vi "Split UDP Data Array.vi"(0 "Array in":string[][](array[string])) -> (1 "Column 1":string[](array[string]), 2 "Column 2":string[](array[string]), 3 "Column 3":string[](array[string]), 4 "Column 4":string[](array[string]))   [LabVIEW 2017]
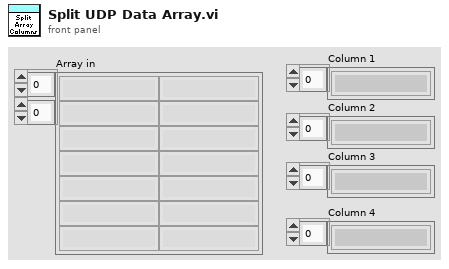
[diagram p1: front panel]
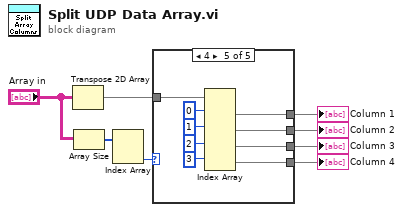
[diagram p0: block diagram]
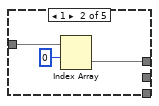
[diagram p3: hidden frame]
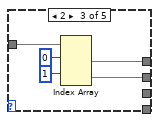
[diagram p4: hidden frame]
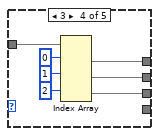
[diagram p5: hidden frame]
diagram:
  n1 = Transpose 2D Array(2D array="Array in") -> (transposed array=w8:string[][])
  n2 = Array Size(array="Array in") -> (size(s)=w6:i32[])
  n3 = Index Array(array=w6) -> (element #2=w5:i32)  [unwired: 2 in, 1 out]
  n4 = case shown="4" w5 {
    tunnel: w8 -> [_ w11 w16 w23 w32]
    tunnel: [_ _ _ _ w27] -> w1
    tunnel: [_ _ _ w17 w26] -> w2
    tunnel: [_ _ w12 w18 w25] -> w3
    tunnel: [_ w9 w13 w19 w24] -> w4
    frame Default {
    }
    frame 1 {
      n5 = Index Array(array=w11, index (row)=0) -> (element=w9:string[])  [unwired: 1 in]
    }
    frame 2 {
      n6 = Index Array(array=w16, index (row) #1=0 ("index (row)"), index (row) #2=1 ("index (row)")) -> (element #1=w13:string[], element #2=w12:string[])  [unwired: 2 in]
    }
    frame 3 {
      n7 = Index Array(array=w23, index (row) #1=0 ("index (row)"), index (row) #2=1 ("index (row)"), index (row) #3=2 ("index (row)")) -> (element #1=w19:string[], element #2=w18:string[], element #3=w17:string[])  [unwired: 3 in]
    }
    frame 4 {
      n8 = Index Array(array=w32, index (row) #1=0 ("index (row)"), index (row) #2=1 ("index (row)"), index (row) #3=2 ("index (row)"), index (row) #4=3 ("index (row)")) -> (element #1=w24:string[], element #2=w25:string[], element #3=w26:string[], element #4=w27:string[])  [unwired: 4 in]
    }
  }
  "Column 1" <- w4
  "Column 2" <- w3
  "Column 3" <- w2
  "Column 4" <- w1
